vi "Set Up Dialog - Microphone.vi"() -> ()   [LabVIEW 2012]
panel:
  in  "Done":bool
  # "iWorx - Microphone - Set Up"
  # "Calibration Instructions"
  # "1. Connect the NI myDAQ to your computer using a USB cable.\n\n2. Connect the MSN-100 microphone to the Audio In port on the NI myDAQ."
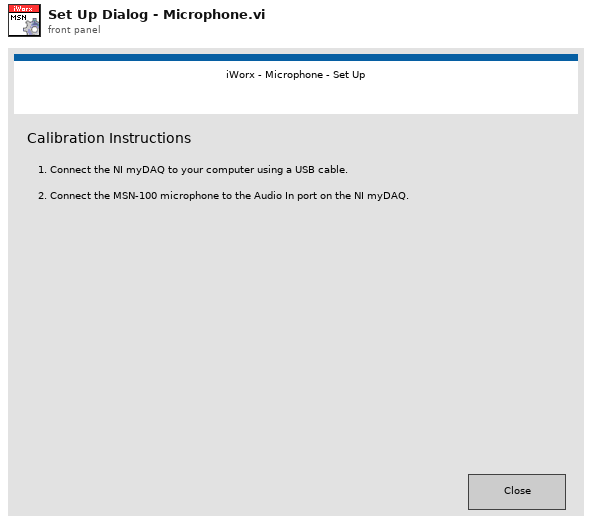
[diagram p1: front panel]
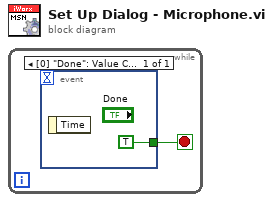
[diagram p0: block diagram]
diagram:
  n1 = while {
    stop <- w1 stop-if-true
    n2 = event shown="[0] \"Done\": Value Change;  Panel Close" {
      selector: _ -> [_]
      dyn-events: _ -> [_]
      timeout: _ -> [_]
      tunnel: [TRUE] -> w1
      event "Done": Value Change; Panel Close {
        n3 = event-data() -> ()  [unwired: 1 in, 1 out]
      }
    }
  }
